vi "distance.vi"(10 "P1":dbl[](array[numeric]), 11 "P2":dbl[](array[numeric])) -> (2 "Dist P1P2":dbl)   [LabVIEW 2018]
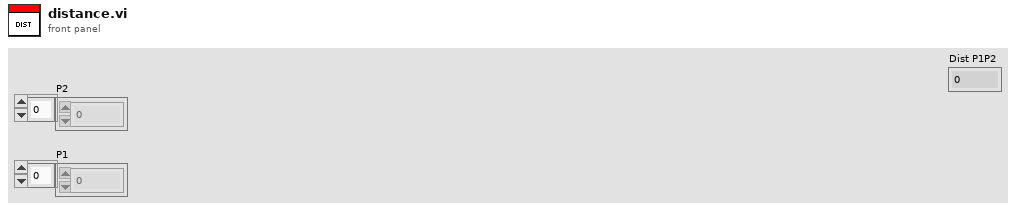
[diagram p1: front panel]
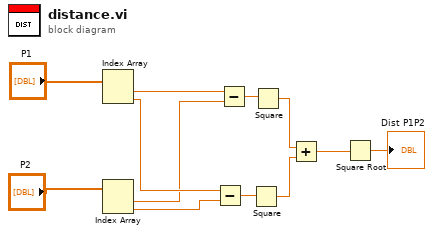
[diagram p0: block diagram]
diagram:
  n1 = Index Array(array="P1") -> (element #1=w2:dbl, element #2=w4:dbl)  [unwired: 2 in]
  n2 = Index Array(array="P2") -> (element #1=w3:dbl, element #2=w5:dbl)  [unwired: 2 in]
  n3 = Subtract(x=w4, y=w5) -> (x-y=w9:dbl)
  n4 = Subtract(x=w2, y=w3) -> (x-y=w8:dbl)
  n5 = Square(x=w9) -> (x^2=w11:dbl)
  n6 = Square(x=w8) -> (x^2=w10:dbl)
  n7 = Add(x=w10, y=w11) -> (x+y=w12:dbl)
  n8 = Square Root(x=w12) -> (sqrt(x)=→"Dist P1P2":dbl)
